vi "Find Workspace.vi"(8 "Error In":errorcluster, 10 "Control In":T2={"I-O.lvclass"=refnum, "Motion.lvclass"=refnum, "Dispenser.lvclass"=refnum}, 11 "Workspace In":refnum<class "Fixture.lvclass">) -> (0 "Error Out":errorcluster, 1 "Workspace Out":T1, 2 "Control Out":T2, 3 "Workspace Out":refnum<class "Fixture.lvclass">)   [LabVIEW 2016, in "Fixture.lvclass"]
uses:
  Fixture.lvclass
  Controller/I-O/I-O.lvclass
  Workspace.ctl
  Controller/Controllers.ctl
  Controller/Controller.lvclass
  Controller/Motion/Motion.lvclass
  Controller/Dispenser/Dispenser.lvclass
  Controller/Motion/A3200/A3200.lvclass
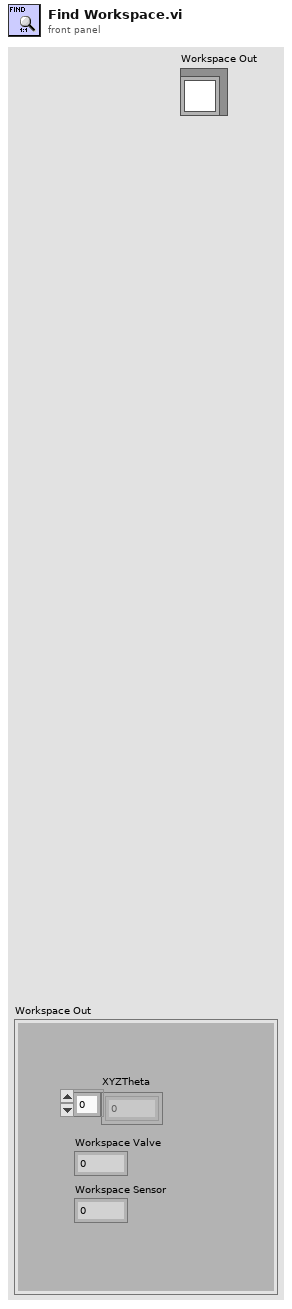
[diagram p1: front panel]
types:
  T1 = typedef "Fixture.lvclass/Workspace.ctl" = cluster{"XYZTheta":dbl[], "Workspace Valve":i32, "Workspace Sensor":i32}
  T2 = typedef "Controller.lvclass/Controllers.ctl" = cluster{"I-O.lvclass":refnum<class "I-O.lvclass">, "Motion.lvclass":refnum<class "Motion.lvclass">, "Dispenser.lvclass":refnum<class "Dispenser.lvclass">}
  T3 = typedef "I-O.lvclass/Pin Map.ctl" = cluster{"Region Valves":i32[], "Extra Valves":dbl[][][], "Tool Primary Valve":i32, "Tool Secondary Valve":i32, "Region Sensors":i32[], "Extra Sensors":dbl[][][], "Tool Primary Sensor":dbl, "Tool Secondary Sensor":dbl, "Compression Sensor":dbl, "5V":i32}
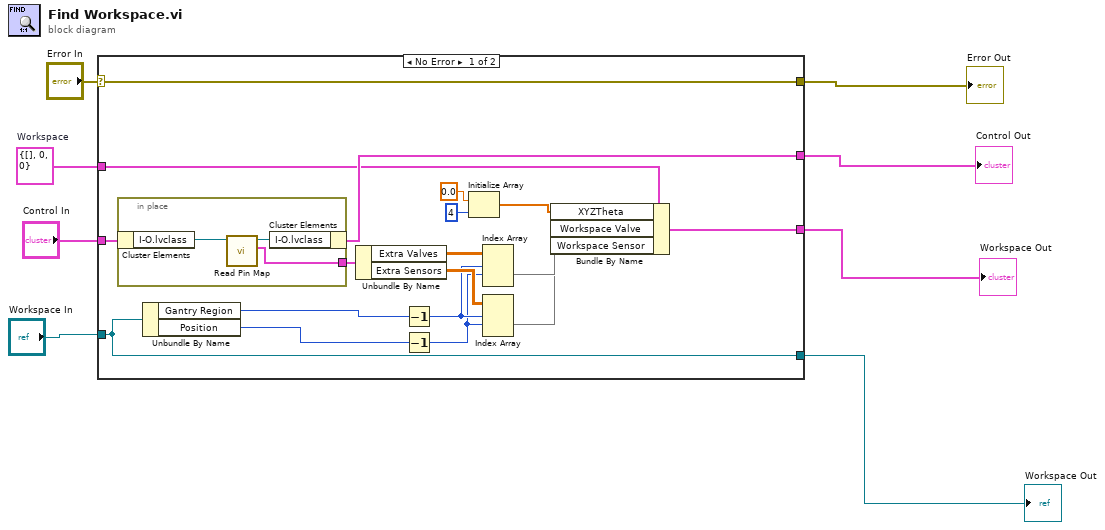
[diagram p0: block diagram]
diagram:
  w4 = T1 {"XYZTheta"=[], "Workspace Valve"=0, "Workspace Sensor"=0}  # Workspace
  n1 = case shown="No Error" "Error In" {
    selector: "Error In" -> [w26 w33]
    tunnel: [w26 w33] -> w7
    tunnel: [w21 w32] -> w5
    tunnel: "Workspace In" -> [w21 w32]
    tunnel: w4 -> [w13 w31]
    tunnel: [w15 w31] -> w3
    tunnel: "Control In" -> [w25 w30]
    tunnel: [w24 w30] -> w1
    frame No Error {
      n2 = in-place {
        in-place-border: [w27] -> w20
        n3 = in-place-cluster #1(w25) -> ("I-O.lvclass"=w29:refnum<class "I-O.lvclass">)
        n4 = call-dynamic "Read Pin Map.vi"("I-O in"=w29) -> ("Pin Map 2"=w27:T3, "I-O out"=w28:refnum<class "I-O.lvclass">)  [unwired: 8 in, 1 out]
        n5 = in-place-cluster #1("I-O.lvclass"=w28) -> (w24:T2)
      }
      n6 = Unbundle By Name(w21) -> ("Gantry Region"=w12:i32, "Position"=w10:i32)
      n7 = Unbundle By Name(w20) -> ("Extra Valves"=w19:dbl[][][], "Extra Sensors"=w18:dbl[][][])
      n8 = Decrement(x=w12) -> (x-1=w11:i32)
      n9 = Decrement(x=w10) -> (x-1=w9:i32)
      n10 = Initialize Array(0.0 ("element"), 4 ("dimension size")) -> (w14:dbl[])
      n11 = Index Array(array=w19, index (dim 0)=w11, index (dim 1)=w9) -> (element=w17:dbl[])  [unwired: 1 in]
      n12 = Index Array(array=w18, index (dim 0)=w11, index (dim 1)=w9) -> (element=w16:dbl[])  [unwired: 1 in]
      n13 = Bundle By Name(cluster=w13, "XYZTheta"=w14, "Workspace Valve"=w17, "Workspace Sensor"=w16) -> (w15:T1)
    }
    frame Error {
    }
  }
  "Error Out" <- w7
  "Workspace Out" <- w5
  "Control Out" <- w1
  "Workspace Out" <- w3
